vi "LAC Cmd000_File Save_Read.vi"(6 "R/W (F:Read)":bool, 7 "timeout(ms)":u32, 8 "error in":errorcluster, 10 "FileNo#":T1(ring), 11 "VISA name in":refnum<visa-resource-name>) -> (0 "error out":errorcluster, 1 "readout":string, 3 "VISA name out":refnum<visa-resource-name>)   [LabVIEW 8.6]
panel:
  # "Choose the file you want to read or to write to."
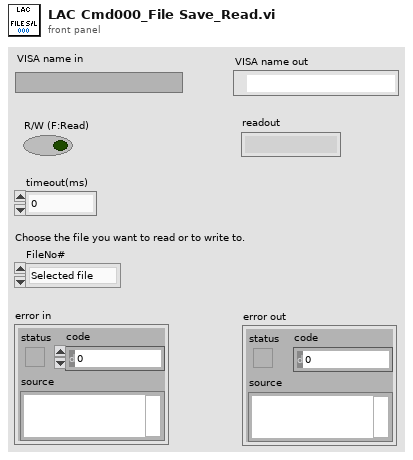
[diagram p1: front panel]
types:
  T1 = enum16{"Selected file", "File 1", "File 2", "File 3", "File 4", "File 5", "File 6"}
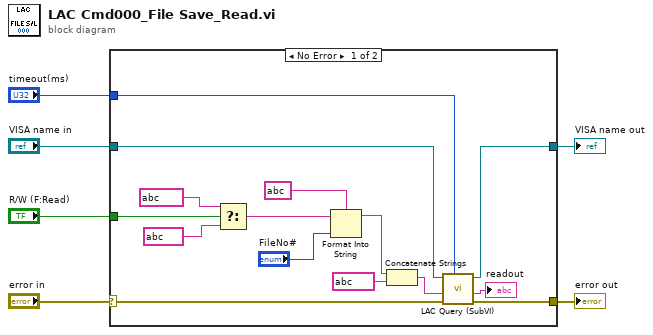
[diagram p0: block diagram]
diagram:
  n1 = case shown="No Error" "error in" {
    selector: "error in" -> [w17 w23]
    tunnel: "VISA name in" -> [w19 w22]
    tunnel: [w21 w22] -> w5
    tunnel: [w20 w23] -> w4
    tunnel: "timeout(ms)" -> [w18 _]
    tunnel: "R/W (F:Read)" -> [w10 _]
    frame #0 {
      n2 = Select(t=string ? ("string"), s=w10, f=string ? ("string")) -> (s? t:f=w9:string)
      n3 = Format Into String(format string=string ?, initial string=w9, "FileNo#") -> (resulting string=w13:string)  [unwired: 1 in, 1 out]
      n4 = Concatenate Strings(w13, string ? ("write buffer")) -> (w15:string)
      n5 = call "LAC Query (SubVI).vi"("timeout(ms)"=w18, "error in"=w17, "Command"=w15, "VISA name in"=w19) -> ("error out"=w20:errorcluster, "read buffer"=→"readout":string, "VISA name out"=w21:refnum<visa-resource-name>)  [unwired: 5 in]
    }
    frame #1 {
    }
  }
  "VISA name out" <- w5
  "error out" <- w4
